vi "VoltageCurrent.vi"(7 "Self-Calibrate at the beginning?":bool, 8 "Range (Volts)":dbl=10.0 format="%.2p", 9 "Resolution in Digits":T1=5.5 items=["3 1/2"=3.5, "4 1/2"=4.5, "5 1/2"=5.5, "6 1/2"=6.5, "7 1/2"=7.5], 10 "Function":T2, 11 "Instrument Descriptor":refnum<k15>) -> (0 "error out":errorcluster, 1 "output array":string[](array[string]), 2 "Measurement (Volts)":dbl format="%_7p", 3 "instrument handle out":refnum<k15>, 5 "Over Range?":bool)   [LabVIEW 2019]
uses:
  <instrlib>/niDMM/nidmm.llb/niDMM Function.ctl
  <instrlib>/niDMM/nidmm.llb/niDMM Resolution in Digits.ctl
  <instrlib>/niDMM/nidmm.llb/niDMM Configure Measurement Digits.vi
panel:
  out "Waveform Chart":dbl(graph)
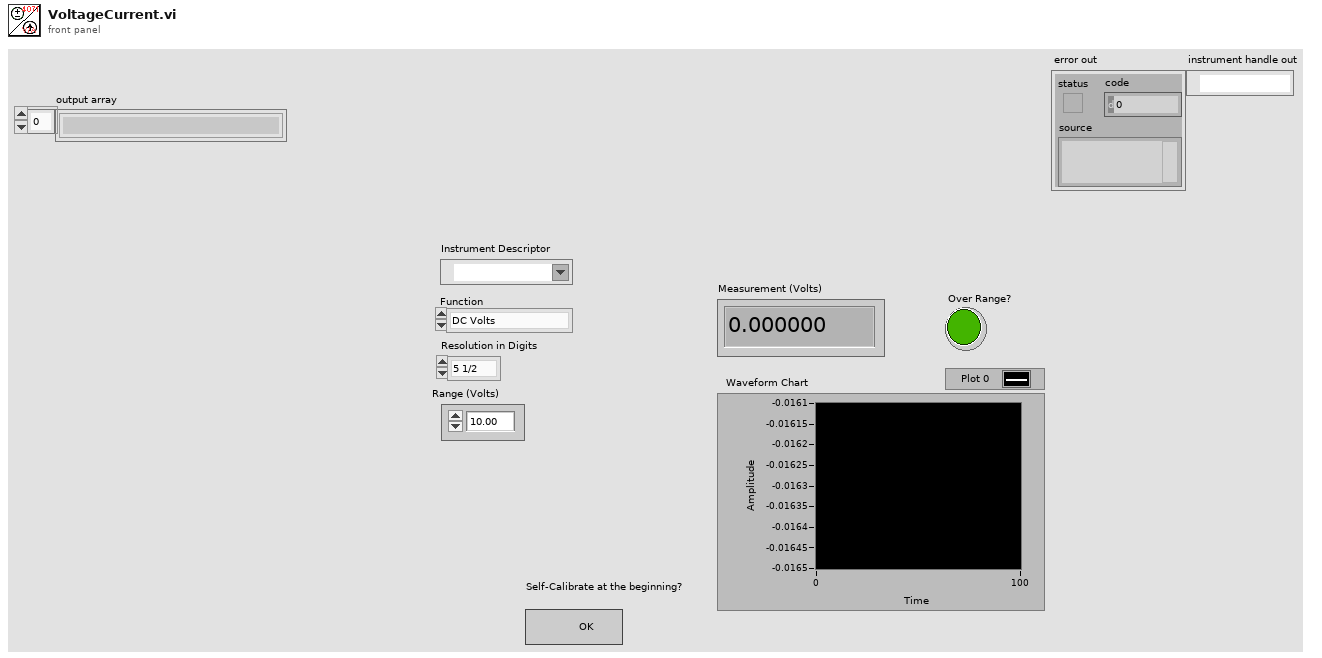
[diagram p1: front panel]
types:
  T1 = typedef "niDMM Resolution in Digits.ctl" = dbl
  T2 = typedef "niDMM Function.ctl" = enum16{"DC Volts", "AC Volts", "DC Current", "AC Current", "2-wire Resistance", "4-wire Resistance", "Diode", "Frequency", "Period", "AC Volts DC Coupled", "Capacitance", "Inductance", "Temperature"}
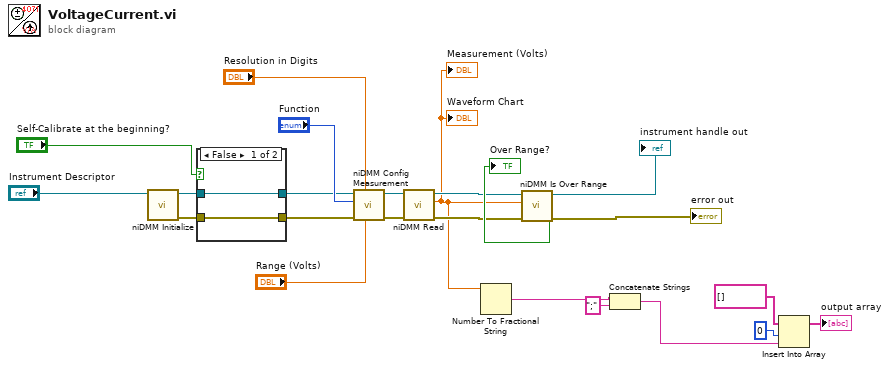
[diagram p0: block diagram]
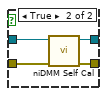
[diagram p2: hidden frame]
diagram:
  n1 = call <instrlib>:"niDMM Initialize.vi"("Instrument Descriptor"="Instrument Descriptor") -> ("error out"=w21:errorcluster, "instrument handle out"=w22:refnum<k15>)  [unwired: 9 in]
  n2 = case shown="False" "Self-Calibrate at the beginning?" {
    tunnel: w22 -> [w25 w29]
    tunnel: w21 -> [w24 w28]
    tunnel: [w24 w27] -> w11
    tunnel: [w25 w26] -> w10
    frame False {
    }
    frame True {
      n3 = call <instrlib>:"niDMM Self Cal.vi"("error in (no error)"=w28, "instrument handle"=w29) -> ("error out"=w27:errorcluster, "instrument handle out"=w26:refnum<k15>)  [unwired: 8 in]
    }
  }
  n4 = call-poly <instrlib>:"niDMM Config Measurement.vi"("Range"="Range (Volts)", "Resolution in Digits"="Resolution in Digits", "error in (no error)"=w11, "Function"="Function", "instrument handle"=w10) -> ("error out"=w15:errorcluster, "instrument handle out"=w14:refnum<k15>)  [unwired: 5 in]
  n5 = call <instrlib>:"niDMM Read.vi"("error in (no error)"=w15, "instrument handle"=w14) -> ("error out"=w17:errorcluster, "Measurement"=w7:dbl, "instrument handle out"=w16:refnum<k15>)  [unwired: 7 in]
  "Measurement (Volts)" <- w7
  "Waveform Chart" <- w7
  n6 = Number To Fractional String(number=w7) -> (F-format string=w6:string)  [unwired: 3 in]
  n7 = call <instrlib>:"niDMM Is Over Range.vi"("error in (no error)"=w17, "Measurement"=w7, "instrument handle"=w16) -> ("error out"=→"error out":errorcluster, "Over Range?"=→"Over Range?":bool, "instrument handle out"=→"instrument handle out":refnum<k15>)  [unwired: 6 in]
  n8 = Concatenate Strings(w6, ";" ("string")) -> (w1:string)
  n9 = Insert Into Array(array=string[] [], index=0, new element=w1) -> (→"output array":string[])
